vi "start_pulse_generation.vi"(0 "VISA resource name":refnum<visa-resource-name>, 1 "Enabled array":bool[](array[boolean]), 2 "Channel Array":i32[](array[numeric]), 3 "Sync source array":i32[](array[numeric]), 11 "error in (no error)":errorcluster, 12 "Delays array":dbl[](array[numeric]), 14 "Widths array":dbl[](array[numeric])) -> (4 "VISA resource name out":refnum<visa-resource-name>, 15 "error out":errorcluster)   [LabVIEW 2019]
uses:
  Configure/Configure Chan Mode (Normal).vi
  Quantum Composers 9000 Series.lvlib
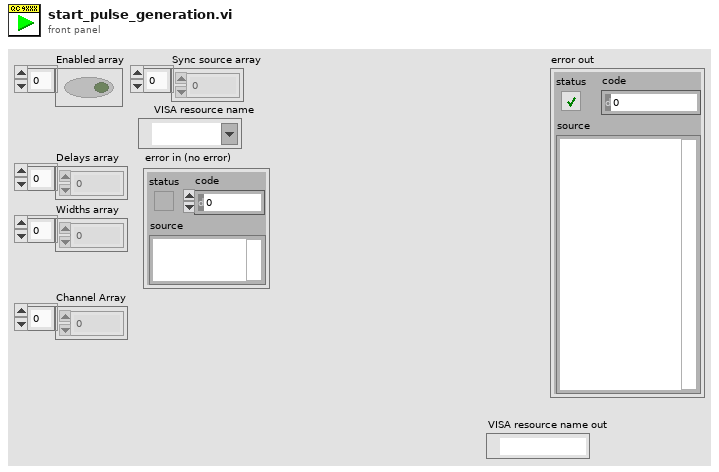
[diagram p1: front panel]
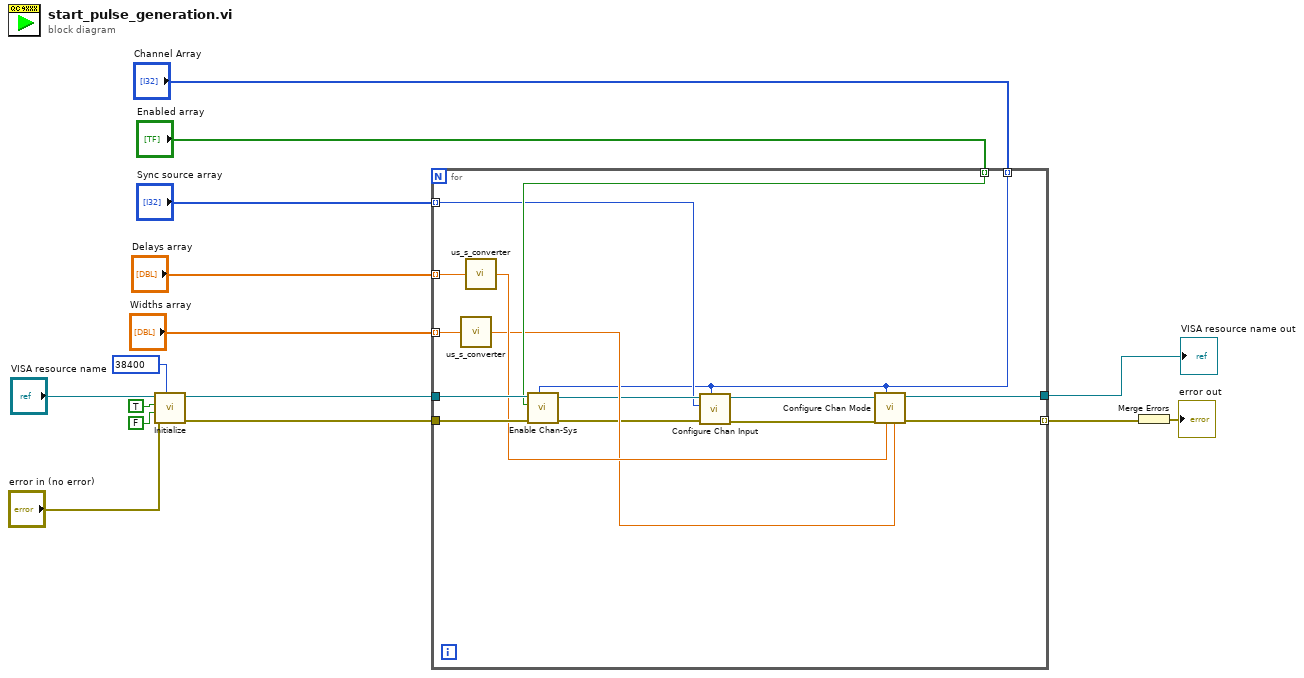
[diagram p0: block diagram]
diagram:
  w1 = u32 38400 items=["4800"=4600, "9600"=9600, "19200"=19200, "38400"=38400, "57600"=57600, "115200"=115200] ("Baud Rate (9600)")
  n1 = call "Initialize.vi"("Baud Rate (9600)"=w1, "error in (no error)"="error in (no error)", "Reset? (T: Yes)"=FALSE, "ID Query? (T: Yes)"=TRUE, "VISA resource name"="VISA resource name") -> ("error out"=w5:errorcluster, "VISA resource name out"=w6:refnum<visa-resource-name>)  [unwired: 5 in]
  n2 = for {
    tunnel: "Channel Array" -> [w18] mode=indexing
    tunnel: "Enabled array" -> [w28] mode=indexing
    tunnel: "Sync source array" -> [w19] mode=indexing
    tunnel: "Delays array" -> [w27] mode=indexing
    tunnel: "Widths array" -> [w26] mode=indexing
    tunnel: w6 -> [w30]
    tunnel: w5 -> [w29]
    tunnel: [w17] -> w2
    tunnel: [w16] -> w4 mode=indexing
    n3 = call "us_s_converter.vi"("Time / us"=w26) -> ("Time / s"=w24:dbl)  [unwired: 4 in]
    n4 = call "us_s_converter.vi"("Time / us"=w27) -> ("Time / s"=w25:dbl)  [unwired: 4 in]
    n5 = call "Enable Chan-Sys.vi"("Channel (1:Chan A)"=w18, "error in (no error)"=w29, "State (T:Enabled)"=w28, "VISA resource name"=w30) -> ("error out"=w22:errorcluster, "VISA resource name out"=w23:refnum<visa-resource-name>)  [unwired: 6 in]
    n6 = call "Configure Chan Input.vi"("Channel (1:Chan A)"=w18, "error in (no error)"=w22, "Sync Source (0:To)"=w19, "VISA resource name"=w23) -> ("error out"=w20:errorcluster, "VISA resource name out"=w21:refnum<visa-resource-name>)  [unwired: 6 in]
    n7 = call-poly "Configure Chan Mode.vi"("Width (10 msec)"=w24, "Delay (10 msec)"=w25, "Channel (1:Chan A)"=w18, "error in (no error)"=w20, "VISA resource name"=w21) -> ("error out"=w16:errorcluster, "VISA resource name out"=w17:refnum<visa-resource-name>)  [unwired: 5 in]
  }
  "VISA resource name out" <- w2
  n8 = Merge Errors(w4) -> (→"error out":errorcluster)
